vi "TabControls.vi"() -> ()   [LabVIEW 2016, in "test_ValueSignal.lvlib"]
uses:
  test_ValueSignal.lvlib
  Helper/HelperVI1.vi
  main/apis/Stimulus/ValueSignalByPathString.vi
  main/apis/Assert/AssertControlValueByPathString.vi
  <vilib>/addons/_JKI Toolkits/Caraya/classes/Assert/Assert Equal Value_Variant.vi
  main/apis/Stimulus/ValueSignalByPathArray.vi
  main/apis/Assert/AssertControlValueByPathArray.vi
  <vilib>/addons/_JKI Toolkits/Caraya/classes/Assert/Assert.lvclass
  <vilib>/addons/_JKI Toolkits/Caraya/classes/Test/Test.lvclass
panel:
  out "error out":errorcluster
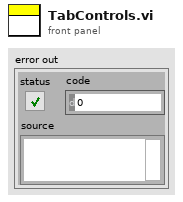
[diagram p1: front panel]
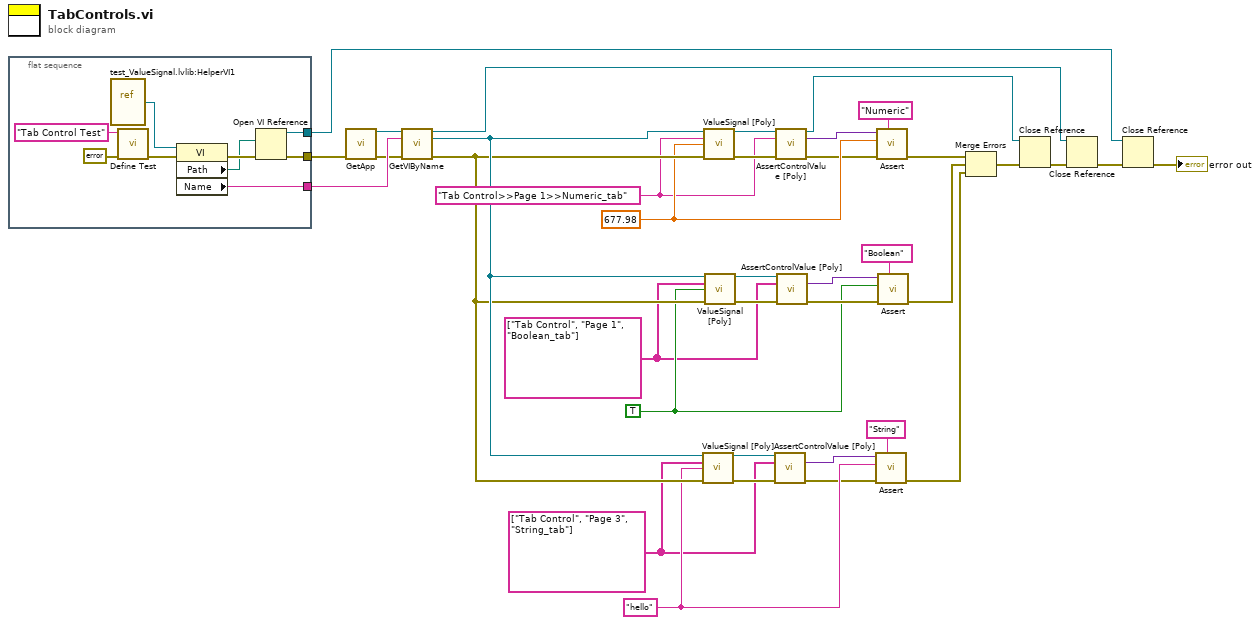
[diagram p0: block diagram]
diagram:
  w1 = string[] ["Tab Control", "Page 1", "Boolean_tab"] ("Class Name")
  w3 = TRUE
  w8 = "Tab Control>>Page 1>>Numeric_tab"
  w13 = 677.98
  w15 = string[] ["Tab Control", "Page 3", "String_tab"] ("Class Name")
  w20 = "hello"
  n1 = flat-sequence {
    tunnel: [w42] -> w33
    tunnel: [w41] -> w35
    tunnel: [w39] -> w32
    frame #0 {
      n2 = vi-ref "test_ValueSignal.lvlib:HelperVI1.vi"() -> (w44:refnum<vi>)
      n3 = call <vilib>:"Define Test.vi"("error in (no error)"=errorcluster {"status"=FALSE, "code"=0, "source"=""}, "Label (VI Title)"="Tab Control Test") -> ("error out"=w45:errorcluster)  [unwired: 9 in]
      n4 = property on="Property Node" class="VI"(reference=w44, error in=w45) -> (error out=w43:errorcluster, "Path"=w40:path, "Name"=w39:string)  [unwired: 1 out]
      n5 = Open VI Reference(vi path=w40, error in (no error)=w43) -> (vi reference=w41:refnum<vi>, error out=w42:errorcluster)  [unwired: 4 in]
    }
  }
  n6 = call "GetApp.vi"("error in (no error)"=w33) -> ("Application Ref"=w34:refnum<vi>, "error out"=w31:errorcluster)  [unwired: 13 in]
  n7 = call "GetVIByName.vi"("Application Ref in"=w34, "VI Name"=w32, "error in (no error)"=w31) -> ("Application Ref out"=w23:refnum<vi>, "VI Reference"=w30:refnum<vi>, "error out"=w22:errorcluster)  [unwired: 10 in]
  n8 = call-poly "ValueSignal [Poly].vi"("VI Reference In"=w30, "Control Path"=w15, "Value (Signaling)"=w20, "error in"=w22) -> ("VI Reference Out"=w19:refnum<vi>, "error out"=w18:errorcluster)  [unwired: 10 in]
  n9 = call-poly "ValueSignal [Poly].vi"("VI Reference In"=w30, "Control Name"=w8, "Value (Signaling)"=w13, "error in"=w22) -> ("VI Reference Out"=w12:refnum<vi>, "error out"=w11:errorcluster)  [unwired: 10 in]
  n10 = call-poly "ValueSignal [Poly].vi"("VI Reference In"=w30, "Control Path"=w1, "Value (Signaling)"=w3, "error in"=w22) -> ("VI Reference Out"=w4:refnum<vi>, "error out"=w5:errorcluster)  [unwired: 10 in]
  n11 = call-poly "AssertControlValue [Poly].vi"("VI Reference In"=w19, "Control Path"=w15, "error in"=w18) -> ("Value"=w16:variant, "error out"=w17:errorcluster)  [unwired: 10 in, 1 out]
  n12 = call-poly "AssertControlValue [Poly].vi"("VI Reference In"=w12, "Control Name"=w8, "error in"=w11) -> ("VI Reference Out"=w25:refnum<vi>, "Value"=w9:variant, "error out"=w10:errorcluster)  [unwired: 10 in]
  n13 = call-poly "AssertControlValue [Poly].vi"("VI Reference In"=w4, "Control Path"=w1, "error in"=w5) -> ("Value"=w7:variant, "error out"=w6:errorcluster)  [unwired: 10 in, 1 out]
  n14 = call-poly <vilib>:"Assert.vi"("Label"="String" ("Label (VI Title)"), "error in (no error)"=w17, "Y"=w20, "X"=w16) -> ("error out"=w27:errorcluster)  [unwired: 7 in]
  n15 = call-poly <vilib>:"Assert.vi"("Label"="Numeric" ("Label (VI Title)"), "error in (no error)"=w10, "Y"=w13, "X"=w9) -> ("error out"=w37:errorcluster)  [unwired: 7 in]
  n16 = call-poly <vilib>:"Assert.vi"("Label"="Boolean" ("Label (VI Title)"), "error in (no error)"=w6, "Y"=w3, "X"=w7) -> ("error out"=w28:errorcluster)  [unwired: 7 in]
  n17 = Merge Errors(w37, w28, w27) -> (w29:errorcluster)
  n18 = Close Reference(reference=w25, error in (no error)=w29) -> (error out=w26:errorcluster)
  n19 = Close Reference(reference=w23, error in (no error)=w26) -> (error out=w24:errorcluster)
  n20 = Close Reference(reference=w35, error in (no error)=w24) -> (error out=→"error out":errorcluster)
